vi "OPEN NEW WORK SHEET.vi"(2 "Sheet?":string="Sheet1", 3 "Excel._Worksheet 2":refnum<k7>, 4 "错误输入（无错误）":errorcluster, 5 "Excel._Workbook":refnum<k7>) -> (0 "错误输出":errorcluster, 1 "Excel._Worksheet":refnum<k7>)   [LabVIEW 2018]
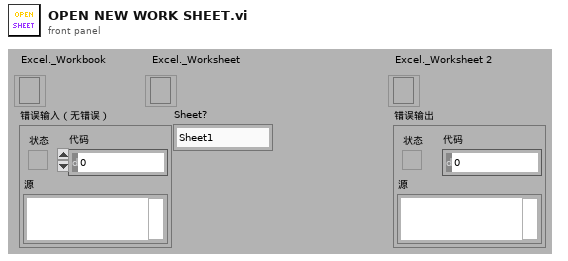
[diagram p1: front panel]
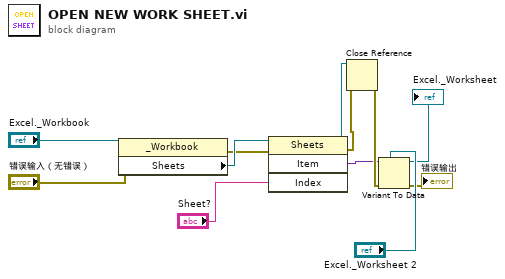
[diagram p0: block diagram]
diagram:
  n1 = property class="_Workbook"(reference="Excel._Workbook", error in="错误输入（无错误）") -> (error out=w9:errorcluster, "Sheets"=w10:refnum<k7>)  [unwired: 1 out]
  n2 = invoke class="Sheets" method="Item"(reference=w10, error in=w9, "Index"="Sheet?") -> (reference out=w8:refnum<k7>, error out=w7:errorcluster, "Item"=w5:variant)  [unwired: 1 in, 1 out]
  n3 = Close Reference(reference=w8, error in (no error)=w7) -> (error out=w6:errorcluster)
  n4 = Variant To Data(error in=w6, type="Excel._Worksheet 2", Variant=w5) -> (data=→"Excel._Worksheet":refnum<k7>, error out=→"错误输出":errorcluster)
